vi "_Parse Power Dynamics Result.vi"(8 "error in (no error)":errorcluster, 10 "Input String":string, 11 "VISA resource name":refnum<visa-resource-name>) -> (0 "error out":errorcluster, 1 "Power Dynamics Results":T1 {"Off Power After" format="%^.3e"; "On Power Peak" format="%^.3e"; "On Power RMS" format="%^.3e"; "Off Power Before" format="%^.3e"}, 2 "Reliability":i32, 3 "VISA resource name out":refnum<visa-resource-name>, 5 "Out Of Tolerance":i32)   [LabVIEW 2020, in "Rohde&Schwarz CMWXP NR FR1 Measurement.lvlib"]
uses:
  <instrlib>/Rohde&Schwarz CMWXP NR FR1 Measurement/Rohde&Schwarz CMWXP NR FR1 Measurement.lvlib
  <instrlib>/Rohde&Schwarz CMWXP NR FR1 Measurement/Private/rsidr_core.llb/rsidr_core.lvlib
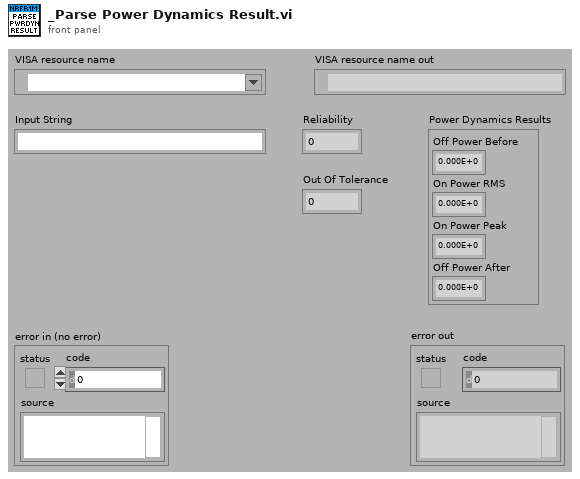
[diagram p1: front panel]
types:
  T1 = cluster{"Off Power Before":dbl, "On Power RMS":dbl, "On Power Peak":dbl, "Off Power After":dbl}
  T2 = cluster{"double array out[0]":dbl, "double array out[1]":dbl, "double array out[2]":dbl, "double array out[3]":dbl}
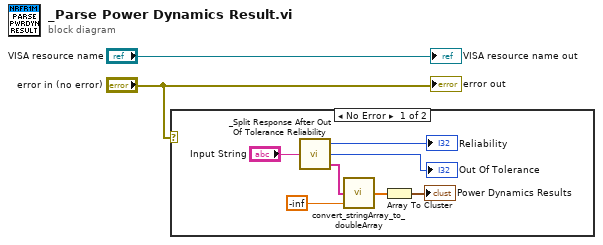
[diagram p0: block diagram]
diagram:
  n1 = case shown="No Error" "error in (no error)" {
    frame No Error {
      n2 = call <instrlib>:"_Split Response After Out Of Tolerance Reliability.vi"("Input String"="Input String") -> ("Reliability out"=→"Reliability":i32, "Out Of Tolerance"=→"Out Of Tolerance":i32, "Response out"=w7:string[])
      n3 = call <instrlib>:"convert_stringArray_to_doubleArray.vi"("default (0)"=-inf, "string array in"=w7) -> ("double array out"=w6:dbl[])  [unwired: 3 in]
      n4 = Array To Cluster(array=w6) -> (cluster=→"Power Dynamics Results":T2)
    }
    frame Error {
    }
  }
  "VISA resource name out" <- "VISA resource name"
  "error out" <- "error in (no error)"
